vi "Flow and Pressure Function Check.vi"(7 "Unit ID (A)":string="A", 8 "error in":errorcluster, 10 "Software Version":u8, 11 "VISA Session In":refnum<visa-resource-name>="Alicat") -> (0 "error out":errorcluster, 1 "Flow Tare Enabled":bool, 2 "Pressure Tare Enabled":bool, 3 "VISA Session Out":refnum<visa-resource-name>)   [LabVIEW 2015]
doc: "Checks to see if pressure tare and flow tare functions are enabled in the devices firmware."
uses:
  <vilib>/Instr/_visa.llb/VISA Flush IO Buffer Mask.ctl
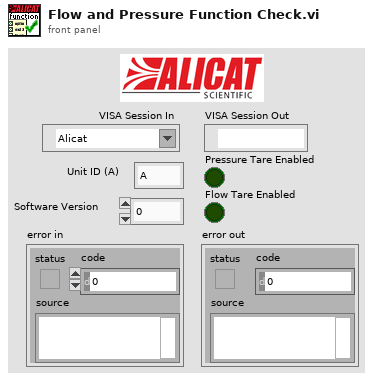
[diagram p1: front panel]
types:
  T1 = typedef "VISA Flush IO Buffer Mask.ctl" = u16
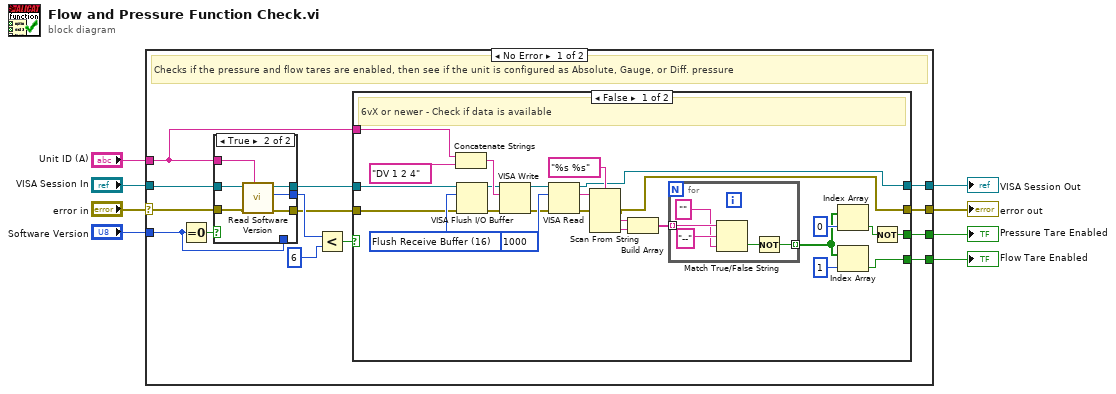
[diagram p0: block diagram]
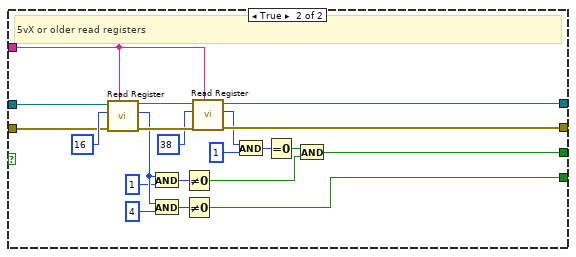
[diagram p2: hidden frame]
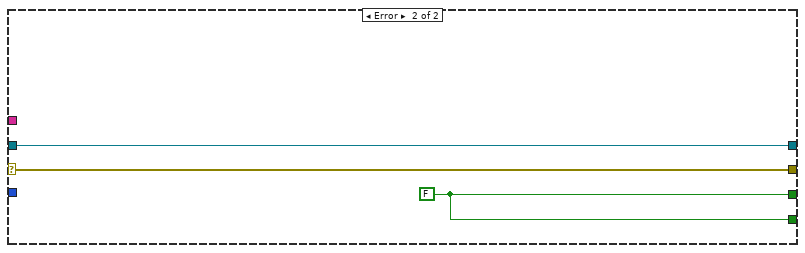
[diagram p4: hidden frame]
diagram:
  n1 = case shown="No Error" "error in" {
    selector: "error in" -> [w14 w84]
    tunnel: [w22 w85] -> w8
    tunnel: [w21 w84] -> w7
    tunnel: "VISA Session In" -> [w13 w85]
    tunnel: "Unit ID (A)" -> [w10 _]
    tunnel: [w20 w83] -> w3
    tunnel: [w19 w83] -> w2
    tunnel: "Software Version" -> [w15 _]
    frame No Error {
      # "Checks if the pressure and flow tares are enabled, then see if the unit is configured as Absolute, Gauge, or Diff. pressure"
      n2 = Equal To 0?(x=w15) -> (x = 0?=w18:bool)
      n3 = case shown="True" w18 {
        tunnel: [w74 w82] -> w12
        tunnel: [w75 w81] -> w11
        tunnel: [w76 w80] -> w17
        tunnel: w15 -> [w76 _]
        tunnel: w14 -> [w74 w79]
        tunnel: w13 -> [w75 w78]
        tunnel: w10 -> [_ w77]
        frame False {
        }
        frame True {
          n4 = call "Read Software Version.vi"("Unit ID (A)"=w77, "error in"=w79, "VISA Session In"=w78) -> ("error out"=w82:errorcluster, "Software Version"=w80:u8, "VISA Session Out"=w81:refnum<visa-resource-name>)  [unwired: 6 in]
        }
      }
      n5 = Less?(x=w17, y=u8 6) -> (x < y?=w9:bool)
      n6 = case shown="False" w9 {
        tunnel: [w27 w73] -> w22
        tunnel: [w28 w72] -> w21
        tunnel: [w24 w59] -> w20
        tunnel: [w31 w58] -> w19
        tunnel: w12 -> [w33 w56]
        tunnel: w11 -> [w32 w55]
        tunnel: w10 -> [w26 w54]
        frame False {
          w42 = T1 16 items=["Flush Receive Buffer"=16, "Write Transmit Buffer to Device"=32, "Flush Receive Buffer (No I/O)"=64, "Flush Transmit Buffer"=128] ("Mask")
          # "6vX or newer - Check if data is available"
          n7 = Concatenate Strings(w26, "DV 1 2 4" ("string")) -> (w46:string)
          n8 = VISA Flush I/O Buffer(VISA resource name=w32, mask (16)=w42, error in (no error)=w33) -> (VISA resource name out=w43:refnum<visa-resource-name>, error out=w44:errorcluster)
          n9 = VISA Write(VISA resource name=w43, write buffer=w46, error in (no error)=w44) -> (VISA resource name out=w40:refnum<visa-resource-name>, error out=w39:errorcluster)  [unwired: 1 out]
          n10 = VISA Read(VISA resource name=w40, byte count=u32 1000, error in (no error)=w39) -> (VISA resource name out=w27:refnum<visa-resource-name>, read buffer=w34:string, error out=w47:errorcluster)  [unwired: 1 out]
          n11 = Scan From String(format string="%s %s", input string=w34, error in=w47) -> (error out=w28:errorcluster, output 1=w37:string, output 2=w36:string)  [unwired: 3 in, 2 out]
          n12 = Build Array(w37, w36) -> (w35:string[])
          n13 = for {
            tunnel: w35 -> [w52] mode=indexing
            tunnel: [w48] -> w25 mode=indexing
            n14 = Match True/False String(2:"", 3:"--" ("false string"), 4:w52) -> (0:w49:bool)  [unwired: 1 out]
            n15 = Not(x=w49) -> (.not. x?=w48:bool)
          }
          n16 = Index Array(array=w25, index=0) -> (element=w23:bool)
          n17 = Index Array(array=w25, index=1) -> (element=w31:bool)
          n18 = Not(x=w23) -> (.not. x?=w24:bool)
        }
        frame True {
          # "5vX or older read registers"
          n19 = call "Read Register.vi"("Unit ID (A)"=w54, "error in"=w56, "Register address"=u16 16, "VISA Session In"=w55) -> ("error out"=w71:errorcluster, "Register Value (I32)"=w67:i32, "VISA Session Out"=w70:refnum<visa-resource-name>)  [unwired: 5 in]
          n20 = And(x=w67, y=1) -> (x .and. y?=w62:i32)
          n21 = And(x=w67, y=4) -> (x .and. y?=w61:i32)
          n22 = Not Equal To 0?(x=w62) -> (x != 0?=w57:bool)
          n23 = Not Equal To 0?(x=w61) -> (x != 0?=w58:bool)
          n24 = call "Read Register.vi"("Unit ID (A)"=w54, "error in"=w71, "Register address"=u16 38, "VISA Session In"=w70) -> ("error out"=w72:errorcluster, "Register Value (I32)"=w53:i32, "VISA Session Out"=w73:refnum<visa-resource-name>)  [unwired: 5 in]
          n25 = And(x=w53, y=1) -> (x .and. y?=w63:i32)
          n26 = Equal To 0?(x=w63) -> (x = 0?=w60:bool)
          n27 = And(x=w60, y=w57) -> (x .and. y?=w59:bool)
        }
      }
    }
    frame Error {
      w83 = FALSE
    }
  }
  "error out" <- w7
  "VISA Session Out" <- w8
  "Pressure Tare Enabled" <- w3
  "Flow Tare Enabled" <- w2
